vi "dispose.vi"(8 "error in":errorcluster, 11 "websocket standalone server in":refnum<class "websocket standalone server.lvclass">) -> (0 "error out":errorcluster)   [LabVIEW 2013, in "websocket standalone server.lvclass"]
uses:
  websocket standalone server.lvclass
  websocket listener message.ctl
  websocket standalone server.lvclass/websocket standalone server.ctl
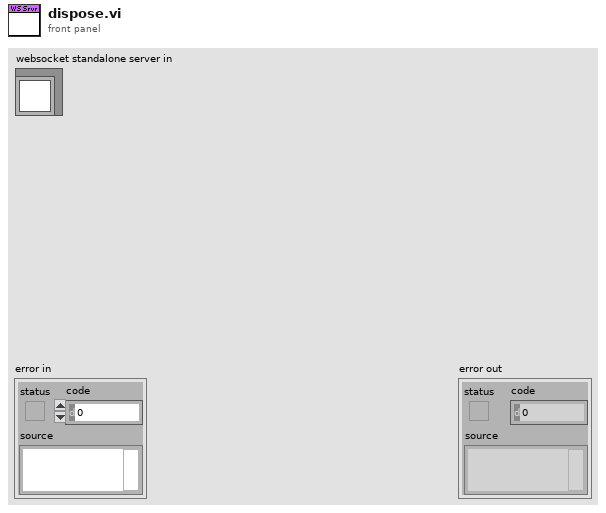
[diagram p1: front panel]
types:
  T1 = typedef "websocket standalone server.lvclass/websocket listener message.ctl" = enum16{"exit", "block socket", "unblock socket"}
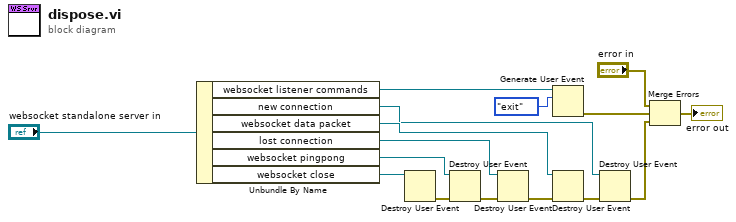
[diagram p0: block diagram]
diagram:
  n1 = Unbundle By Name("websocket standalone server in") -> ("websocket listener commands"=w14:refnum<user-event>, "new connection"=w2:refnum<user-event>, "websocket data packet"=w3:refnum<user-event>, "lost connection"=w4:refnum<user-event>, "websocket pingpong"=w5:refnum<user-event>, "websocket close"=w6:refnum<user-event>)
  n2 = Destroy User Event(user event=w6) -> (error out=w10:errorcluster)  [unwired: 1 in]
  n3 = Destroy User Event(user event=w5, error in=w10) -> (error out=w9:errorcluster)
  n4 = Destroy User Event(user event=w4, error in=w9) -> (error out=w8:errorcluster)
  n5 = Generate User Event(user event=w14, event data cluster=websocket_listener_message."exit" ("element")) -> (error out=w1:errorcluster)  [unwired: 2 in, 1 out]
  n6 = Destroy User Event(user event=w3, error in=w8) -> (error out=w7:errorcluster)
  n7 = Destroy User Event(user event=w2, error in=w7) -> (error out=w15:errorcluster)
  n8 = Merge Errors("error in", w1, w15) -> (→"error out":errorcluster)
